vi "hw2frontend.vi"() -> ()   [LabVIEW 2011]
panel:
  out "Waveform Chart":dbl(graph)
  in  "Boolean":bool
  out "concatenated string":string
  in  "stop":bool
  out "Color Box":u32(colorbox)
  out "Units":string
  in  "Unit Selector":u16(ring) items=["Celsius", "Fahrenheit", "Kelvin"]
  in  "Voltage":dbl(knob) scale=0.0..4.0 scale format="%#.3f"
  out "Temperature":dbl(knob) scale=-350.0..600.0 scale format="%#.3g"
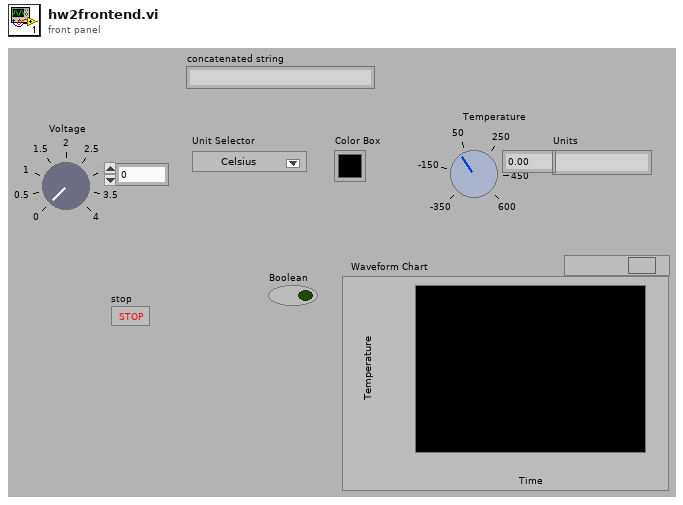
[diagram p1: front panel]
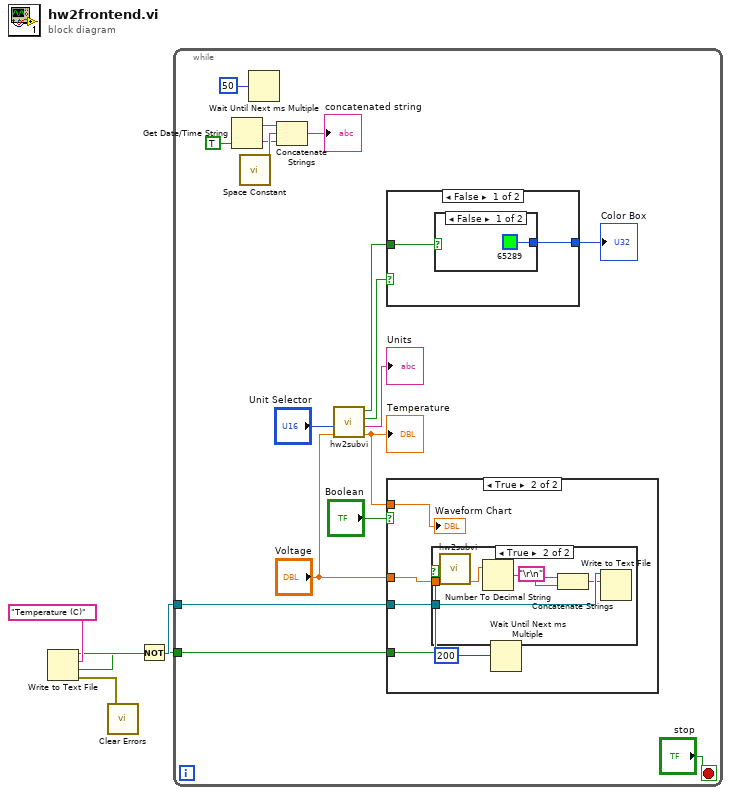
[diagram p0: block diagram]
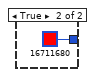
[diagram p4: hidden frame]
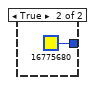
[diagram p5: hidden frame]
diagram:
  n1 = Write to Text File(text="Temperature (C)") -> (refnum out=w4:refnum<file>, cancelled=w3:bool, error out=w1:errorcluster)  [unwired: 3 in]
  n2 = call <vilib>:"Clear Errors.vi"("error in (no error)"=w1) -> ()  [unwired: 6 in, 1 out]
  n3 = Not(x=w3) -> (.not. x?=w2:bool)
  n4 = while {
    tunnel: w4 -> [w8]
    tunnel: w2 -> [w6]
    stop <- "stop" stop-if-true
    n5 = Get Date/Time String(want seconds? (F)=TRUE) -> (date string=w15:string, time string=w13:string)  [unwired: 2 in]
    n6 = call <vilib>:"Space Constant.vi"() -> ("String"=w14:string)
    n7 = Wait Until Next ms Multiple(millisecond multiple=u32 50 ("milliseconds to wait")) -> ()  [unwired: 1 out]
    n8 = Concatenate Strings(w15, w14, w13) -> (→"concatenated string":string)
    n9 = call "hw2subvi.vi"("Voltage"="Voltage", "Unit Selector"="Unit Selector") -> ("Temperature"=w10:dbl, "Units"=→"Units":string, "Input too low"=w21:bool, "Input too high"=w20:bool)  [unwired: 5 in]
    "Temperature" <- w10
    n10 = case shown="False" w21 {
      tunnel: w20 -> [w35 _]
      tunnel: [w34 u32 16775680 ("B")] -> w19
      frame False {
        n11 = case shown="False" w35 {
          tunnel: [u32 65289 ("B") u32 16711680 ("B")] -> w34
          frame False {
          }
          frame True {
          }
        }
      }
      frame True {
      }
    }
    "Color Box" <- w19
    n12 = case shown="True" "Boolean" {
      tunnel: w10 -> [_ w27]
      tunnel: w8 -> [_ w26]
      tunnel: "Voltage" -> [_ w25]
      tunnel: w6 -> [_ w23]
      frame False {
      }
      frame True {
        n13 = case shown="True" w23 {
          tunnel: w26 -> [_ w33]
          tunnel: w25 -> [_ w32]
          frame False {
          }
          frame True {
            n14 = call "hw2subvi.vi"("Voltage"=w32) -> ("Temperature"=w31:dbl)  [unwired: 6 in, 3 out]
            n15 = Number To Decimal String(number=w31) -> (decimal integer string=w29:string)  [unwired: 1 in]
            n16 = Concatenate Strings("\r\n", w29) -> (w28:string)
            n17 = Write to Text File(file (use dialog)=w33, text=w28) -> ()  [unwired: 2 in, 3 out]
          }
        }
        n18 = Wait Until Next ms Multiple(millisecond multiple=u32 200 ("milliseconds to wait")) -> ()  [unwired: 1 out]
        "Waveform Chart" <- w27
      }
    }
  }
